vi "Self-Test.vi"(8 "error in (no error)":errorcluster, 11 "VISA resource name":refnum<visa-resource-name>) -> (0 "error out":errorcluster, 1 "Self-Test Result Message":string, 2 "Self-Test Result Code":i32, 3 "VISA resource name out":refnum<visa-resource-name>)   [LabVIEW 2012, in "Fluke 5080.lvlib"]
doc: "Runs the instrument's self-test routine and returns the test results."
uses:
  <instrlib>/Fluke 5080/Fluke 5080.lvlib
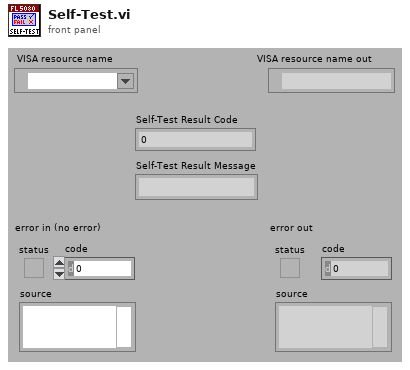
[diagram p1: front panel]
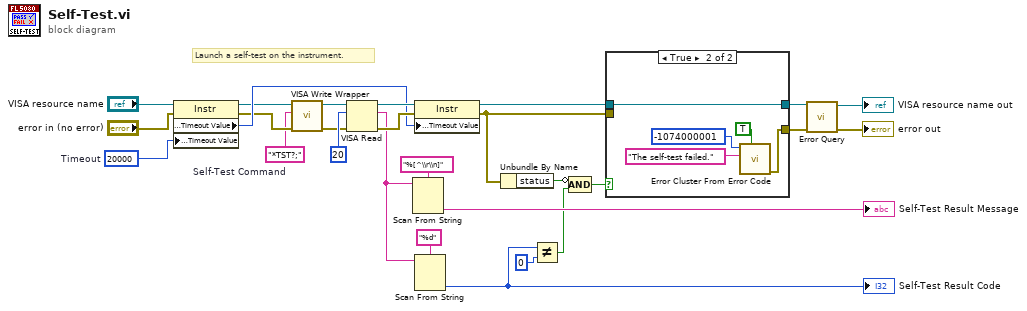
[diagram p0: block diagram]
diagram:
  w16 = u32 20000  # Timeout
  w1 = "*TST?;"  # Self-Test Command
  # "Launch a self-test on the instrument."
  n1 = property class="Instr"(reference="VISA resource name", error in="error in (no error)", "General Settings:Timeout Value"=w16) -> (reference out=w2:refnum<visa-resource-name>, error out=w3:errorcluster, "General Settings:Timeout Value"=w15:u32)
  n2 = call <instrlib>:"VISA Write Wrapper.vi"("error in (no error)"=w3, "Write Buffer"=w1, "VISA resource name"=w2) -> ("error out"=w4:errorcluster, "VISA resource name out"=w5:refnum<visa-resource-name>)  [unwired: 7 out]
  n3 = VISA Read(VISA resource name=w5, byte count=u32 20 ("byte count (20)"), error in (no error)=w4) -> (VISA resource name out=w25:refnum<visa-resource-name>, read buffer=w20:string, error out=w24:errorcluster)  [unwired: 1 out]
  n4 = Scan From String(format string="%[^\\r\\n]" ("Format String"), input string=w20) -> (output 1=→"Self-Test Result Message":string)  [unwired: 2 in, 4 out]
  n5 = property class="Instr"(reference=w25, error in=w24, "General Settings:Timeout Value"=w15) -> (reference out=w14:refnum<visa-resource-name>, error out=w13:errorcluster)
  n6 = Scan From String(format string="%d", input string=w20) -> (output 1=w7:i32)  [unwired: 2 in, 4 out]
  "Self-Test Result Code" <- w7
  n7 = Unbundle By Name(w13) -> ("status"=w9:bool)
  n8 = Not Equal?(x=w7, y=0) -> (x != y?=w10:bool)
  n9 = Compound Arithmetic op=AND(invert w9, w10) -> (w8:bool)
  n10 = case shown="True" w8 {
    tunnel: w14 -> [w29 w34]
    tunnel: w13 -> [w28 _]
    tunnel: [w28 w30] -> w12
    tunnel: [w29 w34] -> w11
    frame False {
    }
    frame True {
      n11 = call <vilib>:"Error Cluster From Error Code.vi"("show call chain? (False)"=TRUE, "error message (\"\")"="The self-test failed." ("Source (VI Name)"), "error code (0)"=-1074000001 ("Code")) -> ("error out"=w30:errorcluster)  [unwired: 1 in, 5 out]
    }
  }
  n12 = call <instrlib>:"Error Query.vi"("error in (no error)"=w12, "VISA resource name"=w11) -> ("error out"=→"error out":errorcluster, "VISA resource name out"=→"VISA resource name out":refnum<visa-resource-name>)  [unwired: 8 out]
